vi "Handle Reply Msg.vi"(8 "error in (no error)":errorcluster, 9 "Panel Controller":refnum<class "Panel Controller Interface.lvclass">, 10 "EditPanel API in":refnum<class "EditPanel API.lvclass">, 11 "Console Reply":refnum<class "Console Reply.lvclass">) -> (0 "error out":errorcluster, 2 "EditPanel API out":refnum<class "EditPanel API.lvclass">)   [LabVIEW 2015, in "EditPanel API.lvlib" / "Console Reply.lvclass"]
uses:
  Console Reply.lvclass
  EditPanel_class/EditPanel API.lvclass
  Panel Control_Interface/Panel_interface/Panel Controller Interface.lvclass
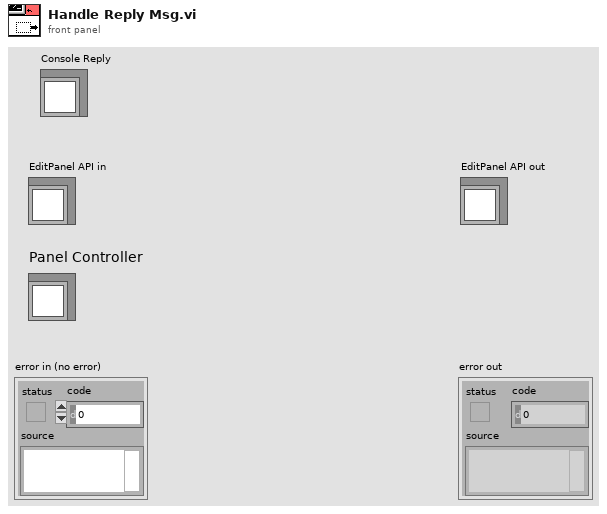
[diagram p1: front panel]
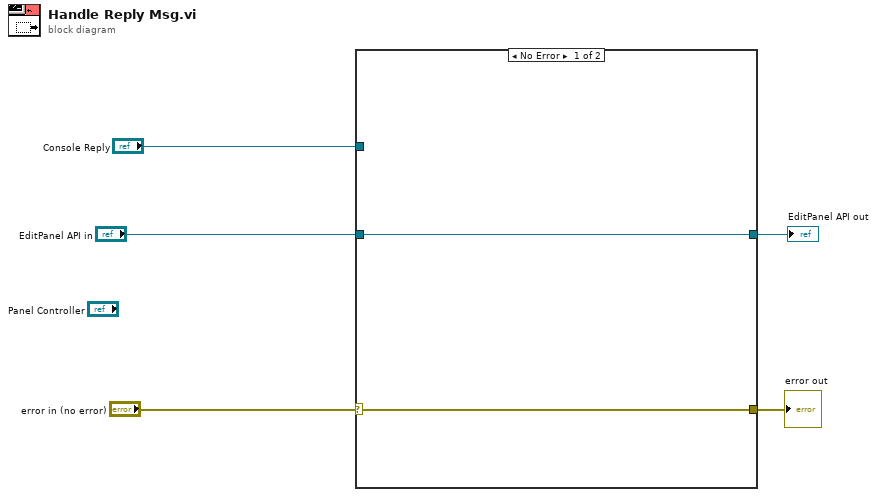
[diagram p0: block diagram]
diagram:
  n1 = case shown="No Error" "error in (no error)" {
    selector: "error in (no error)" -> [w6 w8]
    tunnel: "EditPanel API in" -> [w7 w9]
    tunnel: [w6 w8] -> w4
    tunnel: [w7 w9] -> w3
    tunnel: "Console Reply" -> [_ _]
    frame No Error {
    }
    frame Error {
    }
  }
  "error out" <- w4
  "EditPanel API out" <- w3
